vi "Write Data to File.vi"(8 "error in":errorcluster, 9 "Write?":bool, 10 "Data In":dbl[](array[numeric]), 11 "Neph File Obs in":refnum<class "Neph File Obs.lvclass">) -> (0 "error out":errorcluster, 3 "Neph File Obs out":refnum<class "Neph File Obs.lvclass">)   [LabVIEW 2015, in "Neph File Obs.lvclass"]
uses:
  Neph File Obs.lvclass
  Reusable/File IO/Class/File Observer.lvclass/File Observer.ctl
  Reusable/File IO/Class/File Observer.lvclass
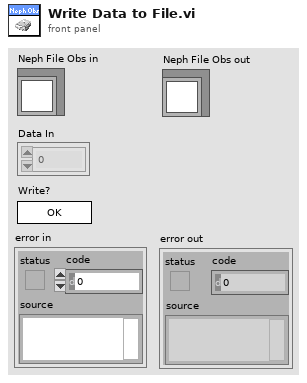
[diagram p1: front panel]
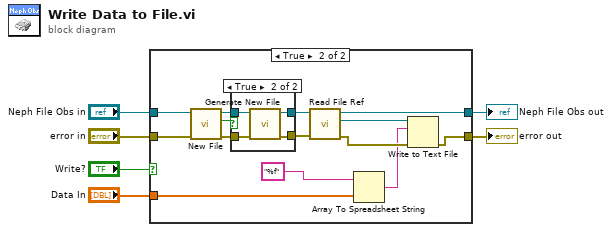
[diagram p0: block diagram]
diagram:
  n1 = case shown="True" "Write?" {
    tunnel: "error in" -> [w7 w22]
    tunnel: [w7 w21] -> w5
    tunnel: "Neph File Obs in" -> [w8 w20]
    tunnel: [w8 w19] -> w3
    tunnel: "Data In" -> [_ w9]
    frame False {
    }
    frame True {
      n2 = call-dynamic "New File.vi"("error in"=w22, "File Observer in"=w20) -> ("error out"=w16:errorcluster, "Exceeded"=w18:bool, "File Observer out"=w17:refnum<class "Neph File Obs.lvclass">)  [unwired: 7 in]
      n3 = case shown="True" w18 {
        tunnel: w17 -> [w24 w28]
        tunnel: w16 -> [w23 w27]
        tunnel: [w24 w26] -> w15
        tunnel: [w23 w25] -> w14
        frame False {
        }
        frame True {
          n4 = call-dynamic "Generate New File.vi"("error in"=w27, "File Obs in"=w28) -> ("error out"=w25:errorcluster, "File Obs out"=w26:refnum<class "Neph File Obs.lvclass">)  [unwired: 7 in, 1 out]
        }
      }
      n5 = call "Read File Ref.vi"("error in"=w14, "File Observer in"=w15) -> ("error out"=w13:errorcluster, "File Ref"=w12:refnum<file>, "File Observer out"=w19:refnum<class "Neph File Obs.lvclass">)  [unwired: 7 in]
      n6 = Array To Spreadsheet String(array=w9, 3:"%f" ("format string")) -> (spreadsheet string=w10:string)  [unwired: 1 in]
      n7 = Write to Text File(file (use dialog)=w12, text=w10, error in=w13) -> (error out=w21:errorcluster)  [unwired: 1 in, 2 out]
    }
  }
  "error out" <- w5
  "Neph File Obs out" <- w3
